vi "Seq Set Power Supply.vi"(8 "Segment Data":T1) -> (0 "Step Hisitory":string[](array[string]), 2 "Segment Data 2":T1)   [LabVIEW 2015]
uses:
  Sequence/type defs/Sequence Info.ctl
  type defs/Power Supply.ctl
panel:
  in  "Set Current Level":dbl
  in  "Set Voltage Level":dbl
  out "String 2":string="Pre Run Station - Glass - Vent Open"
  out "error out":errorcluster
  in  "Description":string
  in  "Save":bool
  in  "Cancel":bool
  # "V（0~15V）"
  # "A（0~30A）"
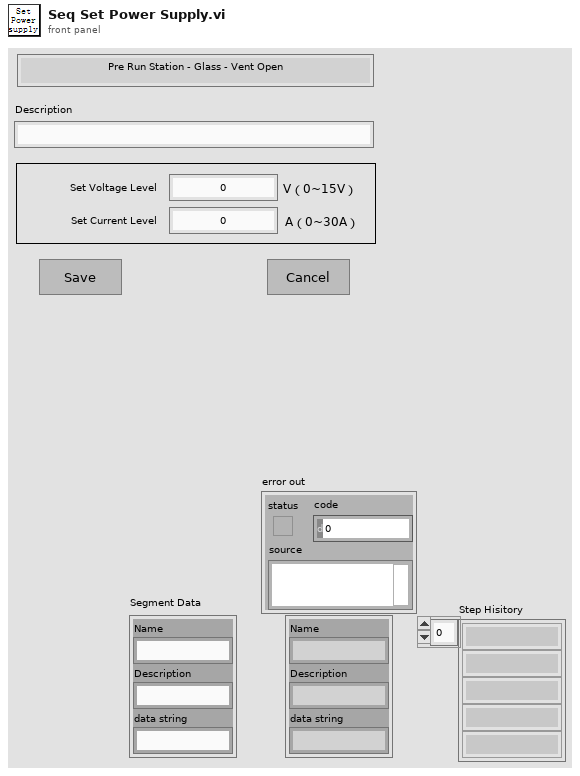
[diagram p1: front panel]
types:
  T1 = typedef "Sequence Info.ctl" = cluster{"Name":string, "Description":string, "data string":string}
  T2 = typedef "Power Supply.ctl" = cluster{"Current":dbl, "Voltage":dbl}
  T3 = cluster{"Segment Data":T1, "Power Supply":T2, "Old Data":string, "New Data":string}
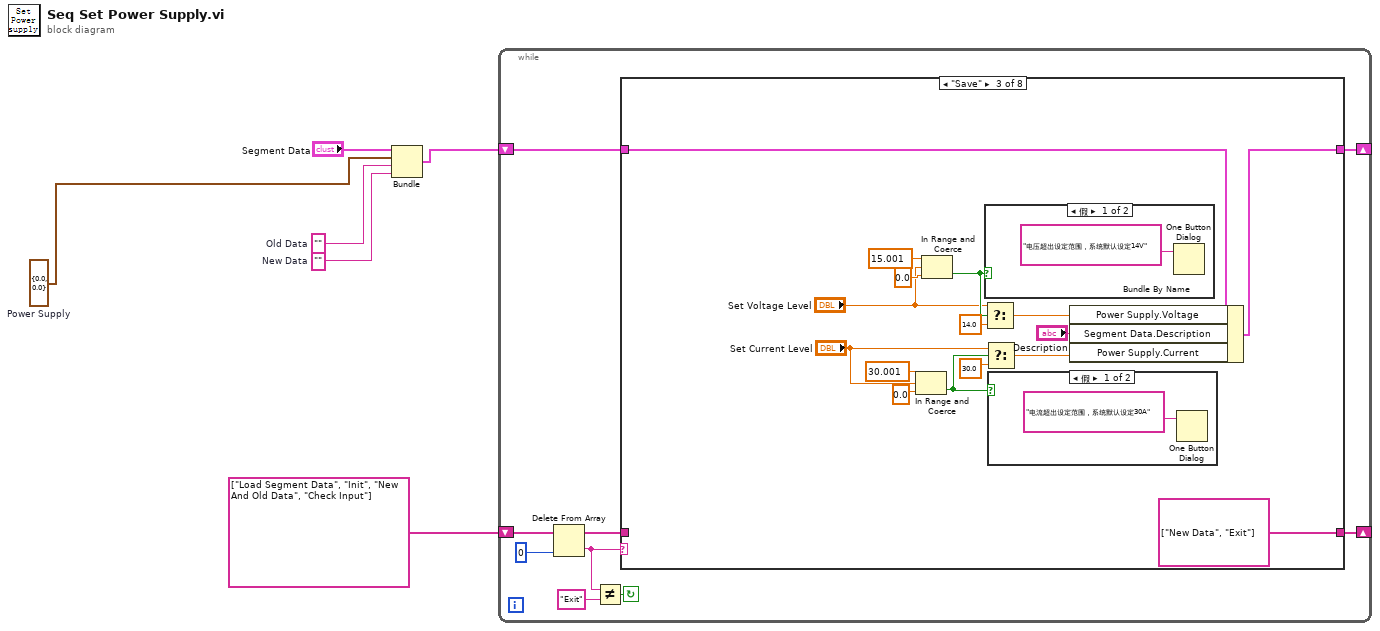
[diagram p0: block diagram]
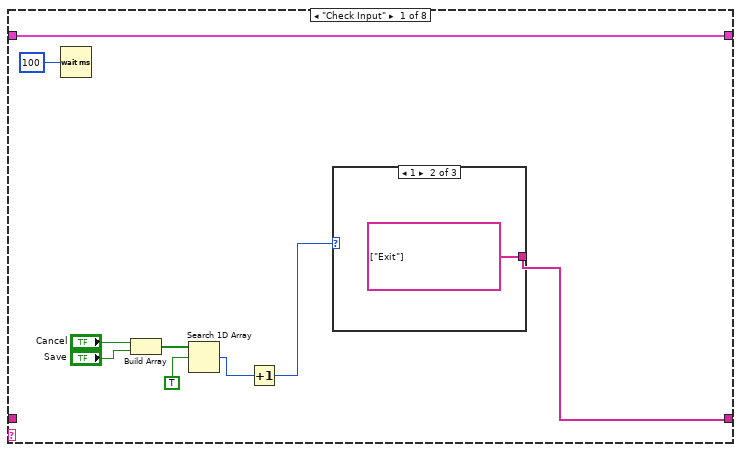
[diagram p2: hidden frame]
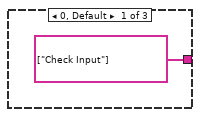
[diagram p3: hidden frame]
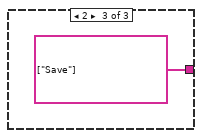
[diagram p4: hidden frame]
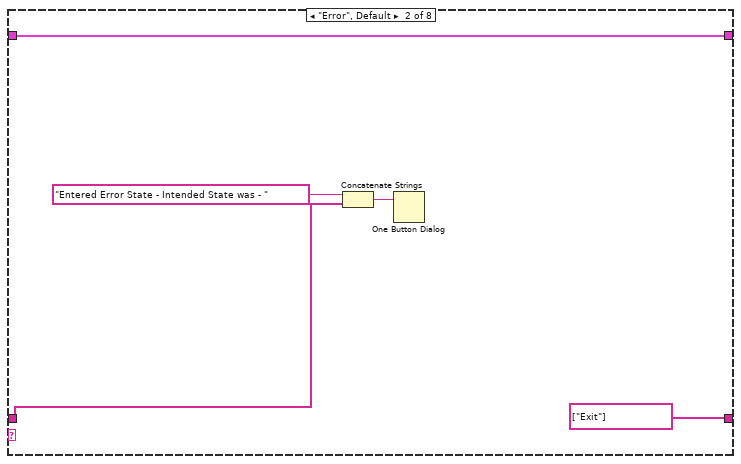
[diagram p5: hidden frame]
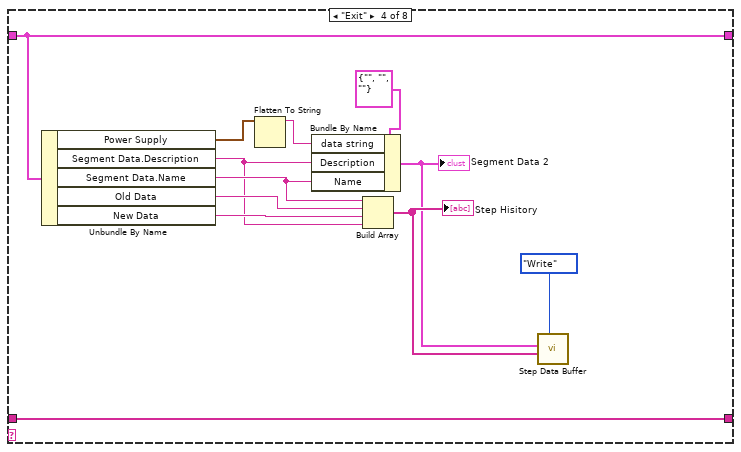
[diagram p8: hidden frame]
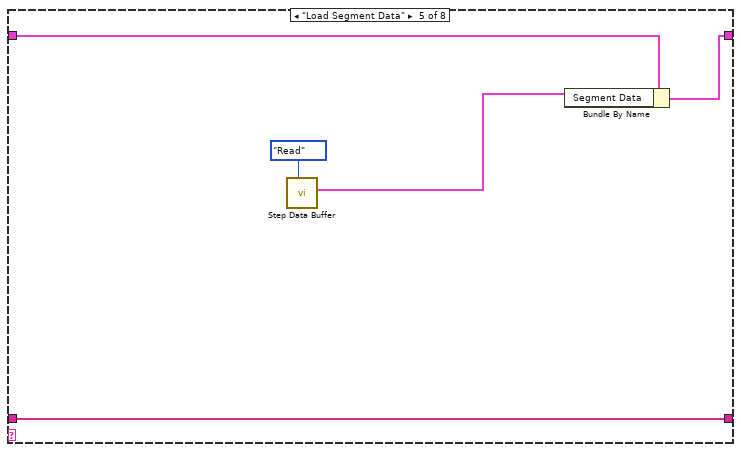
[diagram p9: hidden frame]
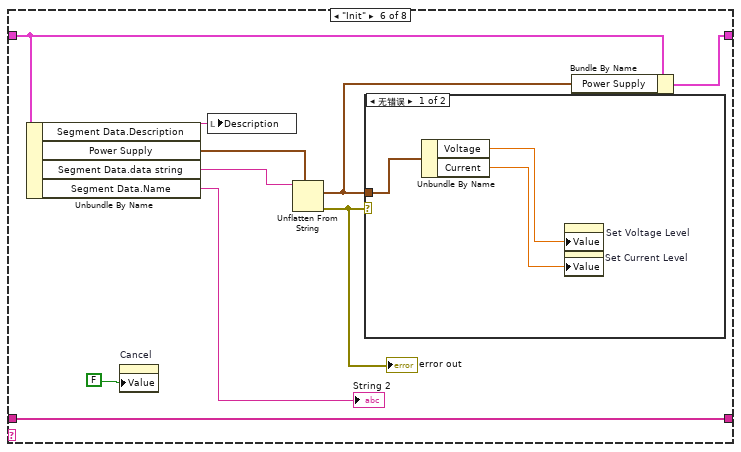
[diagram p10: hidden frame]
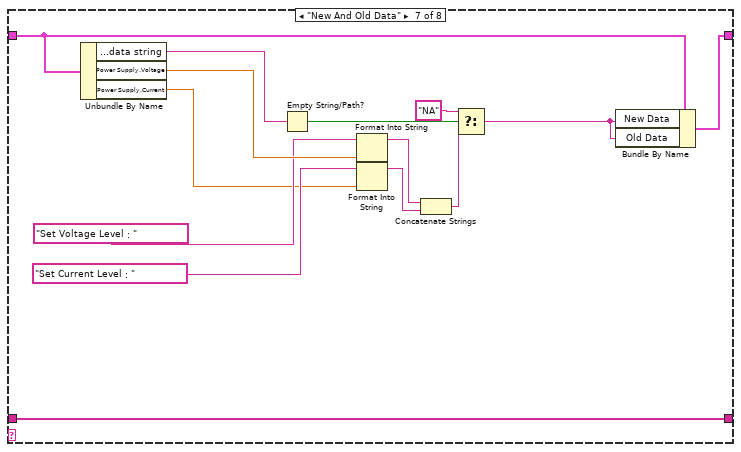
[diagram p12: hidden frame]
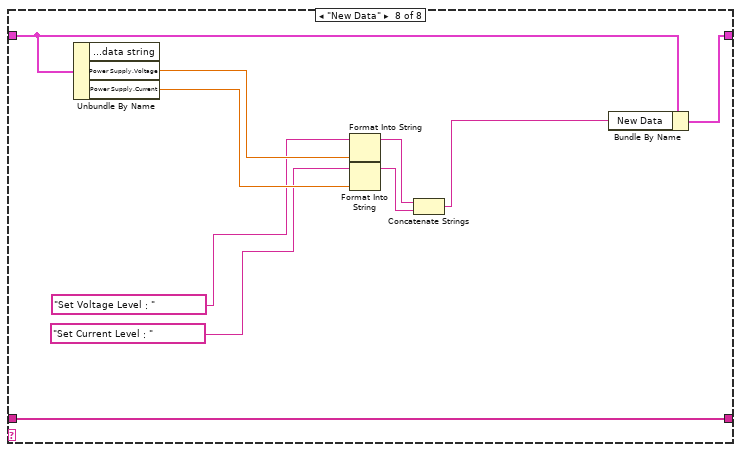
[diagram p13: hidden frame]
diagram:
  w1 = T2 {"Current"=0.0, "Voltage"=0.0}  # Power Supply
  w3 = ""  # New Data
  w4 = ""  # Old Data
  n1 = Bundle("Segment Data"="Segment Data", "Power Supply"=w1, "Old Data"=w4, "New Data"=w3) -> (w5:T3)  [unwired: 1 in]
  n2 = while {
    shift-right: [w15] -> _
    shift-left: string[] ["Load Segment Data", "Init", "New And Old Data", "Check Input"] ("Event queue out") -> [w11]
    shift-right: [w13] -> _
    shift-left: w5 -> [w14]
    stop <- w7 continue-if-true
    n3 = Delete From Array(array=w11, index=0 ("Index")) -> (deleted portion=w9:string, array with subset deleted=w10:string[])  [unwired: 1 in]
    n4 = Not Equal?(x=w9, y="Exit" ("Exit Event")) -> (x != y?=w7:bool)
    n5 = case shown="\"Save\"" w9 {
      tunnel: w10 -> [_ w29 _ w62 w67 w77 w94 w100]
      tunnel: [w16 string[] ["Exit"] ("event queue out") string[] ["New Data", "Exit"] ("Event queue out") w62 w67 w77 w94 w100] -> w15
      tunnel: w14 -> [w19 w32 w47 w55 w64 w70 w83 w99]
      tunnel: [w19 w32 w46 w55 w63 w69 w82 w98] -> w13
      frame "Check Input" {
        n6 = Wait (ms)(milliseconds to wait=u32 100) -> ()  [unwired: 1 out]
        n7 = Build Array("Cancel", "Save") -> (w21:bool[])
        n8 = Search 1D Array(1D array=w21, element=TRUE) -> (index of element=w17:i32)  [unwired: 1 in]
        n9 = Increment(x=w17) -> (x+1=w18:i32)
        n10 = case shown="1" w18 {
          tunnel: [string[] ["Check Input"] ("Events to Insert") string[] ["Exit"] ("Events to Insert") string[] ["Save"] ("Events to Insert")] -> w16
          frame 0, Default {
          }
          frame 1 {
          }
          frame 2 {
          }
        }
      }
      frame "Error", Default {
        n11 = Concatenate Strings("Entered Error State - Intended State was - " ("string"), w29) -> (w30:string)
        n12 = One Button Dialog(message=w30) -> ()  [unwired: 1 in, 1 out]
      }
      frame "Save" {
        n13 = In Range and Coerce(upper limit=30.001 ("上限"), x="Set Current Level", lower limit=0.0 ("下限")) -> (In Range?=w37:bool)  [unwired: 1 out]
        n14 = In Range and Coerce(upper limit=15.001 ("上限"), x="Set Voltage Level", lower limit=0.0 ("下限")) -> (In Range?=w42:bool)  [unwired: 1 out]
        n15 = case shown="假" w42 {
          frame False {
            n16 = One Button Dialog(message="电压超出设定范围，系统默认设定14V" ("消息")) -> ()  [unwired: 1 in, 1 out]
          }
          frame True {
          }
        }
        n17 = Select(t="Set Voltage Level", s=w42, f=14.0 ("t")) -> (s? t:f=w45:dbl)
        n18 = Select(t="Set Current Level", s=w37, f=30.0 ("y")) -> (s? t:f=w33:dbl)
        n19 = case shown="假" w37 {
          frame False {
            n20 = One Button Dialog(message="电流超出设定范围，系统默认设定30A" ("消息")) -> ()  [unwired: 1 in, 1 out]
          }
          frame True {
          }
        }
        n21 = Bundle By Name(cluster=w47, "Power Supply.Voltage"=w45, "Segment Data.Description"="Description", "Power Supply.Current"=w33) -> (w46:T3)
      }
      frame "Exit" {
        n22 = Unbundle By Name(w55) -> ("Power Supply"=w61:T2, "Segment Data.Description"=w51:string, "Segment Data.Name"=w56:string, "Old Data"=w58:string, "New Data"=w57:string)
        n23 = Flatten To String(anything=w61) -> (data string=w59:string)  [unwired: 3 in, 2 out]
        n24 = Bundle By Name(cluster=T1 {"Name"="", "Description"="", "data string"=""} ("Segment Data"), "data string"=w59, "Description"=w51, "Name"=w56) -> (w52:T1)
        "Segment Data 2" <- w52
        n25 = Build Array(w56, w58, w57, w51) -> (w53:string[])
        "Step Hisitory" <- w53
        n26 = call "Step Data Buffer.vi"("Mode"=enum16{"Init", "Read", "Write"}."Write", "Step Hisitory In"=w53, "Segment Data"=w52) -> ()  [unwired: 4 in, 5 out]
      }
      frame "Load Segment Data" {
        n27 = call "Step Data Buffer.vi"("Mode"=enum16{"Init", "Read", "Write"}."Read") -> ("Segment Data"=w65:T1)  [unwired: 6 in, 4 out]
        n28 = Bundle By Name(cluster=w64, "Segment Data"=w65) -> (w63:T3)
      }
      frame "Init" {
        n29 = Unbundle By Name(w70) -> ("Segment Data.Description"=w72:string, "Power Supply"=w75:T2, "Segment Data.data string"=w76:string, "Segment Data.Name"=→"String 2":string)
        n30 = property on="Cancel" class="Bool (严格)"("Value"=FALSE ("Cancel")) -> ()  [unwired: 2 in, 2 out]
        n31 = local write "Description"(w72) -> ()
        n32 = Unflatten From String(type=w75, binary string=w76) -> (value=w71:T2, error out=w74:errorcluster)  [unwired: 3 in, 1 out]
        "error out" <- w74
        n33 = case shown="无错误" w74 {
          tunnel: w71 -> [w80 _]
          frame No Error {
            n34 = Unbundle By Name(w80) -> ("Voltage"=w79:dbl, "Current"=w78:dbl)
            n35 = property on="Set Voltage Level" class="DigNum (严格)"("Value"=w79) -> ()  [unwired: 2 in, 2 out]
            n36 = property on="Set Current Level" class="DigNum (严格)"("Value"=w78) -> ()  [unwired: 2 in, 2 out]
          }
          frame Error {
          }
        }
        n37 = Bundle By Name(cluster=w70, "Power Supply"=w71) -> (w69:T3)
      }
      frame "New And Old Data" {
        n38 = Unbundle By Name(w83) -> ("Segment Data.data string"=w93:string, "Power Supply.Voltage"=w88:dbl, "Power Supply.Current"=w81:dbl)
        n39 = Empty String/Path?(string/path=w93) -> (empty?=w92:bool)
        n40 = Format Into String(initial string="Set Voltage Level：" ("string"), w88) -> (resulting string=w87:string)  [unwired: 2 in, 1 out]
        n41 = Format Into String(initial string="Set Current Level：" ("string"), w81) -> (resulting string=w86:string)  [unwired: 2 in, 1 out]
        n42 = Concatenate Strings(w87, w86) -> (w89:string)
        n43 = Select(t="NA", s=w92, f=w89) -> (s? t:f=w90:string)
        n44 = Bundle By Name(cluster=w83, "New Data"=w90, "Old Data"=w90) -> (w82:T3)
      }
      frame "New Data" {
        n45 = Unbundle By Name(w99) -> ("Power Supply.Voltage"=w104:dbl, "Power Supply.Current"=w102:dbl)  [unwired: 1 out]
        n46 = Format Into String(initial string="Set Voltage Level：" ("string"), w104) -> (resulting string=w103:string)  [unwired: 2 in, 1 out]
        n47 = Format Into String(initial string="Set Current Level：" ("string"), w102) -> (resulting string=w101:string)  [unwired: 2 in, 1 out]
        n48 = Concatenate Strings(w103, w101) -> (w97:string)
        n49 = Bundle By Name(cluster=w99, "New Data"=w97) -> (w98:T3)
      }
    }
  }
